vi "Do.vi"(8 "error in (no error)":errorcluster, 10 "Rival":refnum<class "Peasant.lvclass">, 11 "Weapon in":refnum<class "Weapon.lvclass">) -> (0 "error out":errorcluster, 3 "Weapon out":refnum<class "Weapon.lvclass">)   [LabVIEW 2021, in "Weapon.lvclass"]
uses:
  Weapon.lvclass
  Peasant/Peasant.lvclass
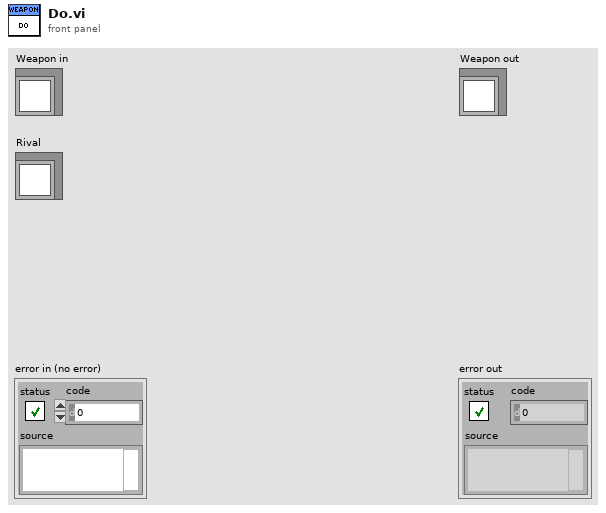
[diagram p1: front panel]
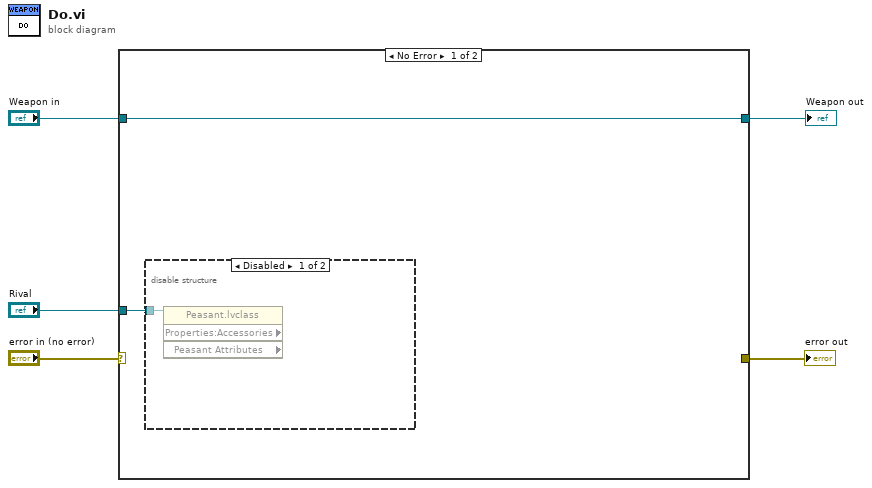
[diagram p0: block diagram]
diagram:
  n1 = case shown="No Error" "error in (no error)" {
    selector: "error in (no error)" -> [_ w10]
    tunnel: [_ w10] -> w4
    tunnel: "Weapon in" -> [w7 w9]
    tunnel: "Rival" -> [w6 _]
    tunnel: [w7 w9] -> w1
    frame No Error {
      n2 = disable-structure shown="Disabled" {
        disable-tunnel: w6 -> [w8 _]
        frame Disabled {
          n3 = property class="Peasant.lvclass" props=["Properties:Accessories", "Peasant Attributes"](reference=w8) -> ()  [unwired: 1 in, 4 out]
        }
        frame Enabled {
        }
      }
    }
    frame Error {
    }
  }
  "error out" <- w4
  "Weapon out" <- w1
